vi "Read Time.vi"(8 "error in (no error)":errorcluster, 11 "FormulaG API in":refnum<class "FormulaG API.lvclass">) -> (0 "error out":errorcluster, 1 "Last Lap":dbl format="%<%M:%S%3u>t", 2 "Current Lap":dbl format="%<%M:%S%3u>t", 3 "FormulaG API out":refnum<class "FormulaG API.lvclass">)   [LabVIEW 2020]
uses:
  Command.ctl
  FormulaG API.lvclass
  <vilib>/IlluminatedG/IG GodotServer/GodotLV/GodotServer/GodotServer.lvclass
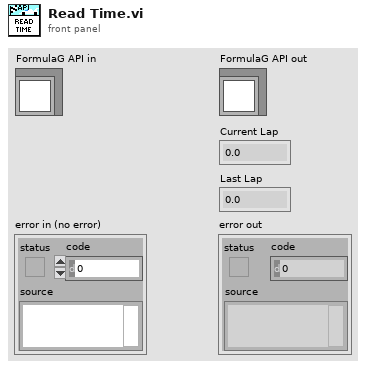
[diagram p1: front panel]
types:
  T1 = enum16{"big-endian, network order", "native, host order", "little-endian"}
  T2 = typedef "FormulaG.lvlib/FormulaG API.lvclass/Command.ctl" = enum8{"None", "Reset Car", "Request State", "Control Car", "Request Info", "Set Options", "Set Camera", "Set Pause", "Request Time"}
  T3 = cluster{"U8":u8, "Current Lap mS":i64, "Last Lap mS":i64}
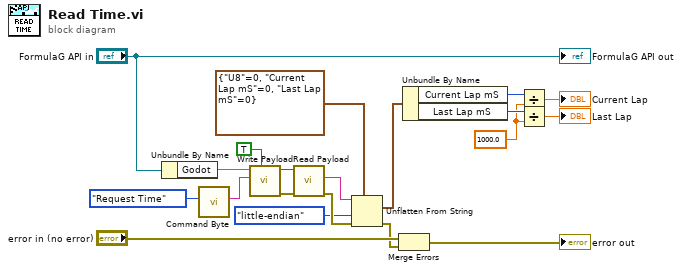
[diagram p0: block diagram]
diagram:
  w6 = 1000.0
  n1 = Unbundle By Name("FormulaG API in") -> ("Godot"=w18)
  n2 = call "Command Byte.vi"("Command"=Command."Request Time") -> ("Command Byte"=w16:string)  [unwired: 10 in]
  n3 = call <vilib>:"Write Payload.vi"("Binary (F = Text)"=TRUE, "Payload"=w16, "GodotServer in"=w18) -> ("error out"=w14:errorcluster, "GodotServer out"=w15:refnum<class "GodotServer.lvclass">)  [unwired: 7 in]
  n4 = call <vilib>:"Read Payload.vi"("error in (no error)"=w14, "GodotServer in"=w15) -> ("error out"=w13:errorcluster, "Payload"=w11:string)  [unwired: 7 in, 1 out]
  n5 = Unflatten From String(type=T3 {"U8"=0, "Current Lap mS"=0, "Last Lap mS"=0}, binary string=w11, byte order (0:big-endian, network order)=T1."little-endian", error in (no error)=w13) -> (value=w9:T3, error out=w2:errorcluster)  [unwired: 1 in, 1 out]
  n6 = Merge Errors("error in (no error)", w2) -> (→"error out":errorcluster)
  n7 = Unbundle By Name(w9) -> ("Current Lap mS"=w8:i64, "Last Lap mS"=w7:i64)
  n8 = Divide(x=w8, y=w6) -> (x/y=→"Current Lap":dbl)
  n9 = Divide(x=w7, y=w6) -> (x/y=→"Last Lap":dbl)
  "FormulaG API out" <- "FormulaG API in"
